vi "update_framescan.vi"(8 "error in (no error)":errorcluster, 9 "config cluster":T1={"DDS board initialization parameters"={"Bypass PLL"=FALSE, "PLL Range"=TRUE, "Update Clock"=FALSE, "Triangle "=FALSE, "SDO Active"=FALSE, "LSB First"=FALSE, "OSK Int"=FALSE, "Output Shaped Keying Enable"=TRUE, "Bypass Sinc"=FALSE, "Digital Part"=TRUE, "OutPut DAC"=TRUE, "Control DAC"=TRUE, "Comparator"=FALSE, "Modus"=0, "Multiplier Value"=15}, "OSK select"=TRUE, "inverse?"="normal", "AOD equilibration time"=0.0, "AOD amplitude"=0, "AOD center frequency"=0.0, "AOD Bandwidth"=0.0} {"DDS board initialization parameters"."Modus" scale=0.0..4.0}, 10 "settings cluster":T4={"number of pixels"=0, "maximum bit-depth"=0, "AOD center freq. (Hz)"=0.0, "AOD bandwidth freq. (Hz)"=0.0, "AOD amplitude"=0.0, "pixel dwell time"=0.0, "AOD equilibration time"=0.0, "x resolution"=0, "y resolution"=0, "z angle (rotation angle, phi)"=0.0, "x angle (tilting angle, phi)"=-1.0, "zoom"=-1.0, "channel offsets"={"channel 0"=0, "channel 1"=0, "channel 2"=0, "channel 3"=0}, "offset (Hz)"=[], "gates"=[], "enable clocks?"=FALSE}, 11 "FPGA VI Reference In":T3) -> (0 "error out":errorcluster)   [LabVIEW 2010]
doc: "This one is doing an update"
uses:
  FPGAWrapperMH120124FrameScan_PXI7813R/settings_cluster_framescan.ctl
  common_typedefs/channels_cluster.ctl
  fpgaVIsAndControls/gate_cluster.ctl
  common_typedefs/gate_parameters_cluster.ctl
  FPGAWrapperMH120124FrameScan_PXI7813R/FPGA_framescan_reference.ctl
  FPGAWrapperMH120124FrameScan_PXI7813R/configuration_cluster_framescan.ctl
  fpgaVIsAndControls/DDS_board_init_cluster.ctl
  <vilib>/rvi/interface/nirviReadWriteControl/nirviReadWriteControl.xnode
  <vilib>/rvi/interface/common/niFpgaNodeNameForErrorReporting.ctl
  <vilib>/rvi/errors/niLvFpgaWhatHappensToTopLevelVI.ctl
  <vilib>/Utility/error.llb/Error Cluster From Error Code.vi
  <vilib>/rvi/errors/niLvFpgaAdjustHostInterfaceError.vi
  NiFpgaLv.dll
panel:
  # "FSK"
  # "Ramped"
  # "FSK"
  # "Chirp Modus"
  # "Unramped"
  # "BPSK"
  # "Single Tone"
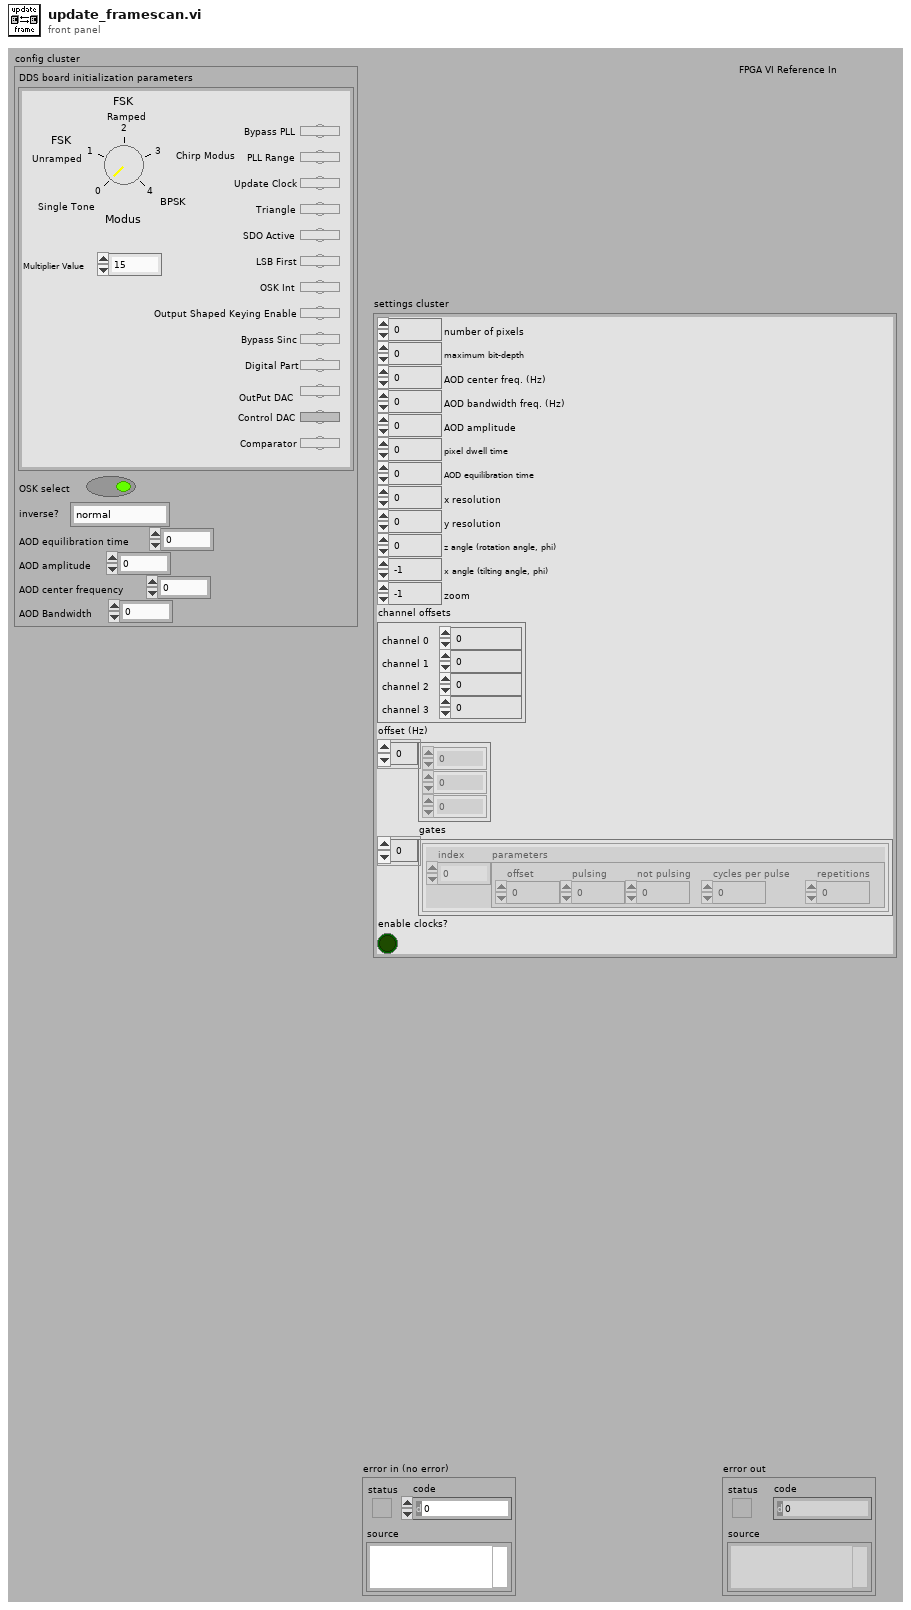
[diagram p1: front panel]
types:
  T1 = typedef "configuration_cluster_framescan.ctl" = cluster{"DDS board initialization parameters":T2, "OSK select":bool, "inverse?":string, "AOD equilibration time":dbl, "AOD amplitude":u16, "AOD center frequency":dbl, "AOD Bandwidth":dbl}
  T2 = typedef "DDS_board_init_cluster.ctl" = cluster{"Bypass PLL":bool, "PLL Range":bool, "Update Clock":bool, "Triangle ":bool, "SDO Active":bool, "LSB First":bool, "OSK Int":bool, "Output Shaped Keying Enable":bool, "Bypass Sinc":bool, "Digital Part":bool, "OutPut DAC":bool, "Control DAC":bool, "Comparator":bool, "Modus":u8, "Multiplier Value":u8}
  T3 = typedef "FPGA_framescan_reference.ctl" = refnum<k20>
  T4 = typedef "settings_cluster_framescan.ctl" = cluster{"number of pixels":i32, "maximum bit-depth":i8, "AOD center freq. (Hz)":dbl, "AOD bandwidth freq. (Hz)":dbl, "AOD amplitude":dbl, "pixel dwell time":dbl, "AOD equilibration time":dbl, "x resolution":i32, "y resolution":i32, "z angle (rotation angle, phi)":dbl, "x angle (tilting angle, phi)":dbl, "zoom":dbl, "channel offsets":T5, "offset (Hz)":dbl[], "gates":T6[], "enable clocks?":bool}
  T5 = typedef "channels_cluster.ctl" = cluster{"channel 0":u32, "channel 1":u32, "channel 2":u32, "channel 3":u32}
  T6 = typedef "gate_cluster.ctl" = cluster{"index":i32, "parameters":T7}
  T7 = typedef "gate_parameters_cluster.ctl" = cluster{"offset":i64, "pulsing":i64, "not pulsing":i64, "cycles per pulse":i64, "repetitions":i64}
  T8 = typedef "niFpgaNodeNameForErrorReporting.ctl" = enum16{"Open FPGA VI Reference", "Read/Write Control", "Invoke Method: Abort", "Invoke Method: Acknowledge IRQ", "Invoke Method: Download", "Invoke Method: FIFO.Configure", "Invoke Method: FIFO.Read", "Invoke Method: FIFO.Start", "Invoke Method: FIFO.Stop", "Invoke Method: FIFO.Write", "Invoke Method: Reset", "Invoke Method: Run", "Invoke Method: Wait on IRQ", "Close FPGA VI Reference"}
  T9 = typedef "niLvFpgaWhatHappensToTopLevelVI.ctl" = enum16{"top level VI scripted behind XNode", "top level VI inlined behind XNode"}
  T10 = cluster{"AOD Bandwidth_x (Hz)":fxp<+/-,36,32>, "AOD Bandwidth_y (Hz)":fxp<+/-,36,32>, "sin Phi":fxp<+/-,36,2>, "cos Phi":fxp<+/-,36,2>, "Bandwidth for LUTs (256pts)":fxp<+,36,0>, "AOD_Amplitude in":u16, "AOD center frequ. (Hz)_x":fxp<+/-,36,32>, "AOD center frequ. (Hz)_y":fxp<+/-,36,32>, "x offset (Hz)":fxp<+/-,36,32>, "y offset (Hz)":fxp<+/-,36,32>}
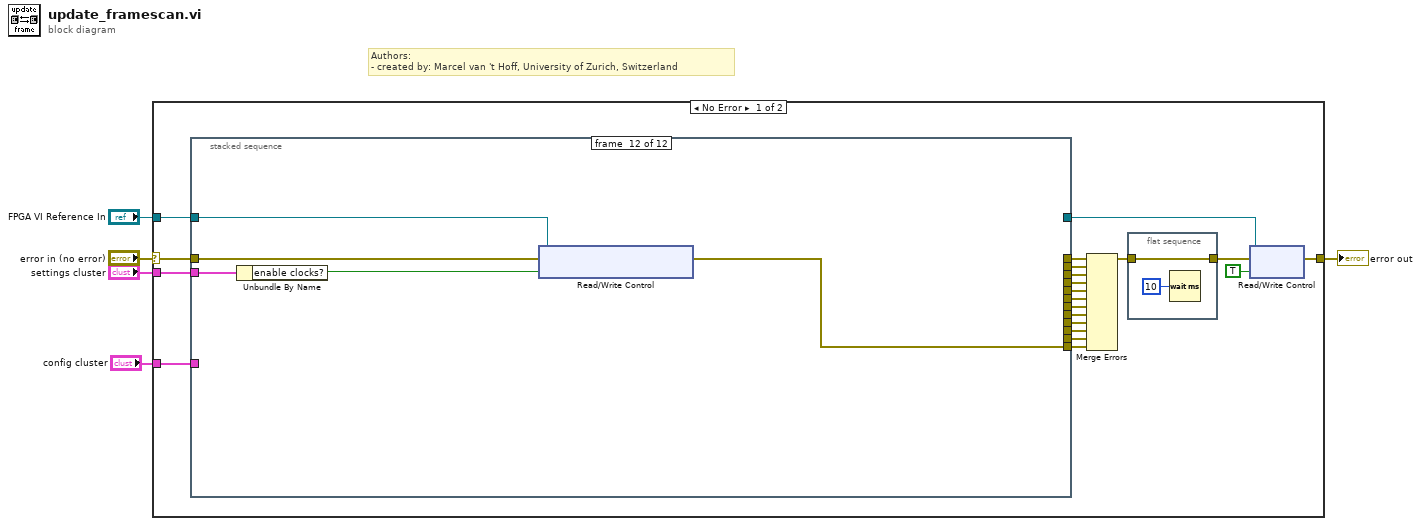
[diagram p0: block diagram]
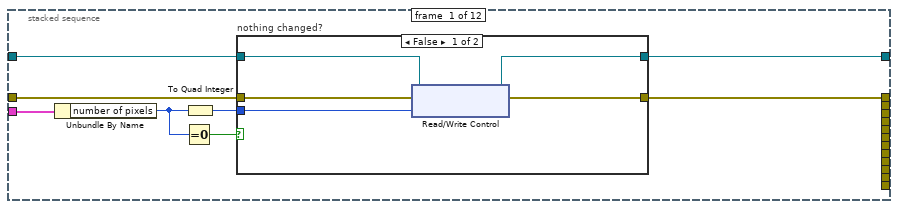
[diagram p2: hidden frame]
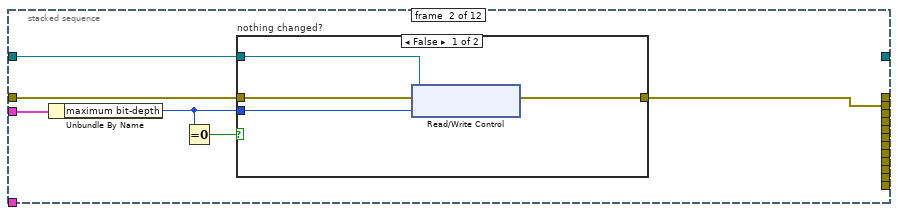
[diagram p4: hidden frame]
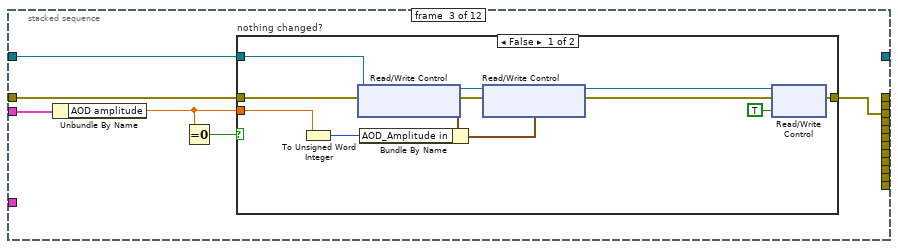
[diagram p6: hidden frame]
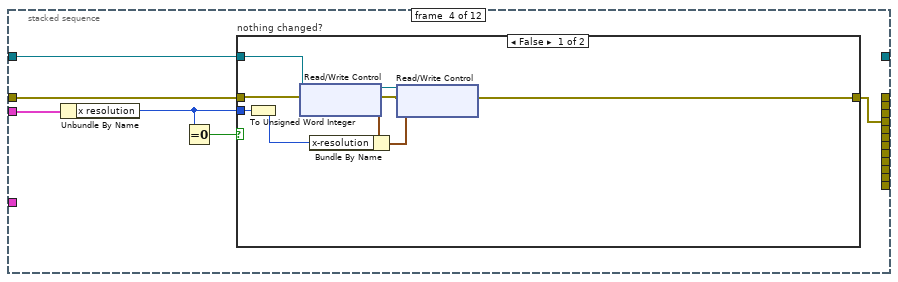
[diagram p8: hidden frame]
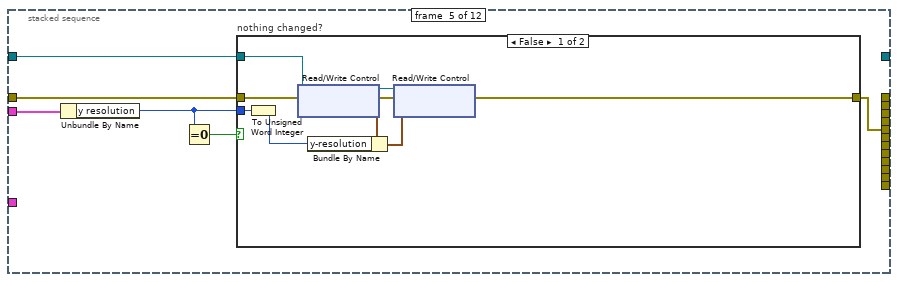
[diagram p10: hidden frame]
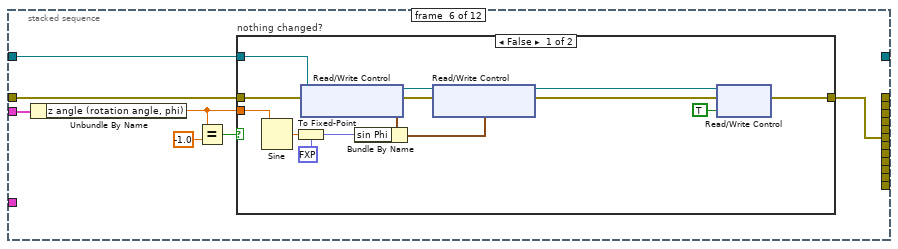
[diagram p12: hidden frame]
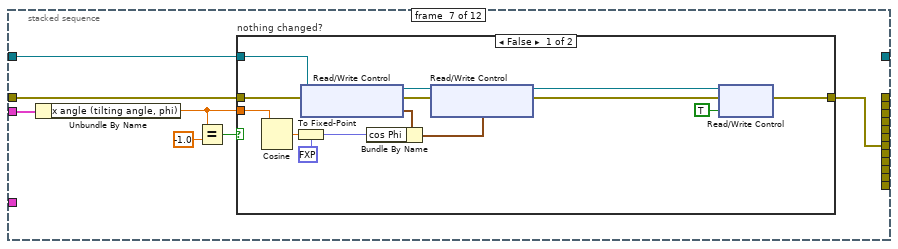
[diagram p14: hidden frame]
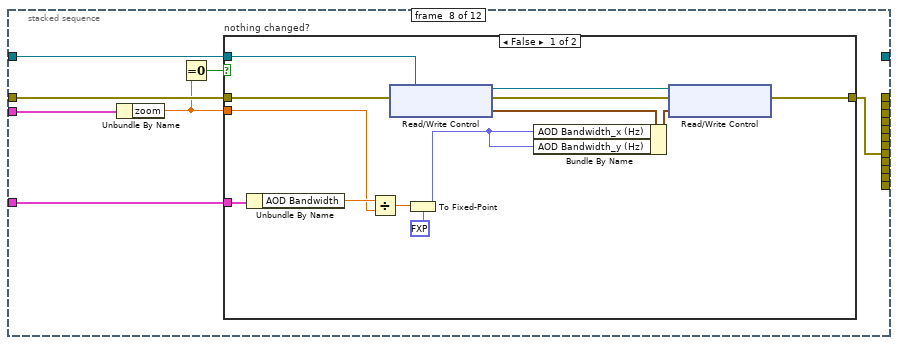
[diagram p16: hidden frame]
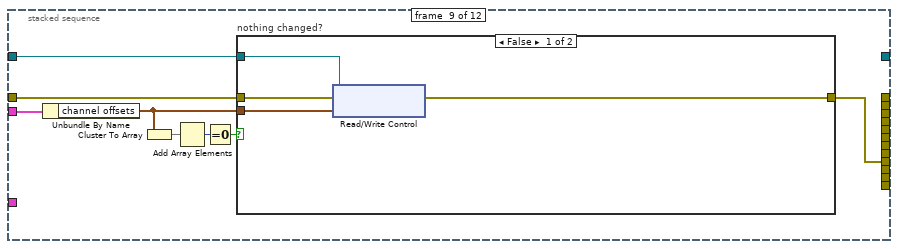
[diagram p18: hidden frame]
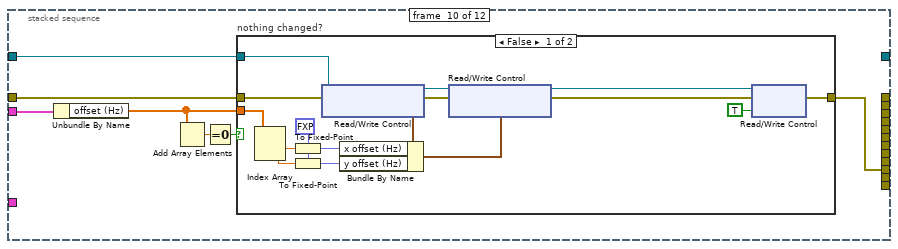
[diagram p20: hidden frame]
diagram:
  # "Authors: \n- created by: Marcel van 't Hoff, University of Zurich, Switzerland"
  n1 = case shown="No Error" "error in (no error)" {
    selector: "error in (no error)" -> [w13 w1389]
    tunnel: "settings cluster" -> [w12 _]
    tunnel: "FPGA VI Reference In" -> [w14 _]
    tunnel: [w25 w1389] -> w3
    tunnel: "config cluster" -> [w7 _]
    frame No Error {
      n2 = stacked-sequence {
        tunnel: w12 -> [w34 w91 w140 w292 w403 w515 w670 w825 w941 w997 w1152 w1308]
        tunnel: [w28 _ _ _ _ _ _ _ _ _ _ _] -> w15
        tunnel: w13 -> [w30 w89 w138 w290 w401 w514 w669 w824 w940 w996 w1149 w1307]
        tunnel: w14 -> [w29 w88 w137 w289 w400 w513 w668 w823 w939 w995 w1150 w1306]
        tunnel: [_ w86 _ _ _ _ _ _ _ _ _ _] -> w16
        tunnel: [_ _ w135 _ _ _ _ _ _ _ _ _] -> w17
        tunnel: [_ _ _ w287 _ _ _ _ _ _ _ _] -> w18
        tunnel: [_ _ _ _ w398 _ _ _ _ _ _ _] -> w19
        tunnel: [_ _ _ _ _ w509 _ _ _ _ _ _] -> w20
        tunnel: [_ _ _ _ _ _ w664 _ _ _ _ _] -> w21
        tunnel: [_ _ _ _ _ _ _ w820 _ _ _ _] -> w22
        tunnel: [_ _ _ _ _ _ _ _ w934 _ _ _] -> w23
        tunnel: [_ _ _ _ _ _ _ _ _ w991 _ _] -> w24
        tunnel: [w27 _ _ _ _ _ _ _ _ _ _ _] -> w10
        tunnel: [_ _ _ _ _ _ _ _ _ _ w1148 _] -> w9
        tunnel: w7 -> [_ _ _ _ _ _ _ w819 _ _ _ _]
        tunnel: [_ _ _ _ _ _ _ _ _ _ _ w1305] -> w6
        frame #0 {
          n3 = Unbundle By Name(w34) -> ("number of pixels"=w33:i32)
          n4 = Equal To 0?(x=w33) -> (x = 0?=w32:bool)
          n5 = To Quad Integer(1:w33) -> (0:w31:i64)
          n6 = case "nothing changed?" shown="False" w32 {
            tunnel: w31 -> [w37 _]
            tunnel: [w39 w85] -> w28
            tunnel: w30 -> [w38 w85]
            tunnel: w29 -> [w36 w84]
            tunnel: [w35 w84] -> w27
            frame False {
              n7 = xnode "Read/Write Control"("FPGA VI Reference In"=w36, "error in"=w38, "number of pixels"=w37) -> ("FPGA VI Reference Out"=w35:T3, "error out"=w39:errorcluster)
            }
            frame True {
              # "nothing changed"
            }
          }
        }
        frame #1 {
          n8 = Unbundle By Name(w91) -> ("maximum bit-depth"=w87:i8)
          n9 = Equal To 0?(x=w87) -> (x = 0?=w90:bool)
          n10 = case "nothing changed?" shown="False" w90 {
            tunnel: w87 -> [w93 _]
            tunnel: [w95 w134] -> w86
            tunnel: w89 -> [w94 w134]
            tunnel: w88 -> [w92 _]
            frame False {
              n11 = xnode "Read/Write Control"("FPGA VI Reference In"=w92, "error in"=w94, "maximum bit depth"=w93) -> ("error out"=w95:errorcluster)  [unwired: 1 out]
            }
            frame True {
              # "nothing changed"
            }
          }
        }
        frame #2 {
          n12 = Unbundle By Name(w140) -> ("AOD amplitude"=w136:dbl)
          n13 = Equal To 0?(x=w136) -> (x = 0?=w139:bool)
          n14 = case "nothing changed?" shown="False" w139 {
            tunnel: [w145 w286] -> w135
            tunnel: w138 -> [w150 w286]
            tunnel: w137 -> [w152 _]
            tunnel: w136 -> [w148 _]
            frame False {
              n15 = To Unsigned Word Integer(number=w148) -> (unsigned 16bit integer=w147:u16)
              n16 = xnode "Read/Write Control"("FPGA VI Reference In"=w152, "error in"=w150) -> ("FPGA VI Reference Out"=w151:T3, "error out"=w149:errorcluster, "FPGA parameters"=w142:T10)
              n17 = Bundle By Name(cluster=w142, "AOD_Amplitude in"=w147) -> (w141:T10)
              n18 = xnode "Read/Write Control"("FPGA VI Reference In"=w151, "error in"=w149, "FPGA parameters"=w141) -> ("FPGA VI Reference Out"=w144:T3, "error out"=w146:errorcluster)
              n19 = xnode "Read/Write Control"("FPGA VI Reference In"=w144, "error in"=w146, "reset in"=TRUE) -> ("error out"=w145:errorcluster)  [unwired: 1 out]
            }
            frame True {
              # "nothing changed"
            }
          }
        }
        frame #3 {
          n20 = Unbundle By Name(w292) -> ("x resolution"=w288:i32)
          n21 = Equal To 0?(x=w288) -> (x = 0?=w291:bool)
          n22 = case "nothing changed?" shown="False" w291 {
            tunnel: [w295 w397] -> w287
            tunnel: w290 -> [w298 w397]
            tunnel: w289 -> [w297 _]
            tunnel: w288 -> [w301 _]
            frame False {
              n23 = To Unsigned Word Integer(number=w301) -> (unsigned 16bit integer=w296:u16)
              n24 = xnode "Read/Write Control"("FPGA VI Reference In"=w297, "error in"=w298) -> ("FPGA VI Reference Out"=w293:T3, "error out"=w294:errorcluster, "scan settings"=w300:cluster{"x-resolution":u16, "y-resolution":u16})
              n25 = Bundle By Name(cluster=w300, "x-resolution"=w296) -> (w299:cluster{"x-resolution":u16, "y-resolution":u16})
              n26 = xnode "Read/Write Control"("FPGA VI Reference In"=w293, "error in"=w294, "scan settings"=w299) -> ("error out"=w295:errorcluster)  [unwired: 1 out]
            }
            frame True {
              # "nothing changed"
            }
          }
        }
        frame #4 {
          n27 = Unbundle By Name(w403) -> ("y resolution"=w399:i32)
          n28 = Equal To 0?(x=w399) -> (x = 0?=w402:bool)
          n29 = case "nothing changed?" shown="False" w402 {
            tunnel: [w408 w508] -> w398
            tunnel: w401 -> [w410 w508]
            tunnel: w400 -> [w411 _]
            tunnel: w399 -> [w412 _]
            frame False {
              n30 = To Unsigned Word Integer(number=w412) -> (unsigned 16bit integer=w405:u16)
              n31 = xnode "Read/Write Control"("FPGA VI Reference In"=w411, "error in"=w410) -> ("FPGA VI Reference Out"=w407:T3, "error out"=w409:errorcluster, "scan settings"=w406:cluster{"x-resolution":u16, "y-resolution":u16})
              n32 = Bundle By Name(cluster=w406, "y-resolution"=w405) -> (w404:cluster{"x-resolution":u16, "y-resolution":u16})
              n33 = xnode "Read/Write Control"("FPGA VI Reference In"=w407, "error in"=w409, "scan settings"=w404) -> ("error out"=w408:errorcluster)  [unwired: 1 out]
            }
            frame True {
              # "nothing changed"
            }
          }
        }
        frame #5 {
          n34 = Unbundle By Name(w515) -> ("z angle (rotation angle, phi)"=w512:dbl)
          n35 = Equal?(x=w512, y=-1.0) -> (x = y?=w511:bool)
          n36 = case "nothing changed?" shown="False" w511 {
            tunnel: [w519 w663] -> w509
            tunnel: w514 -> [w524 w663]
            tunnel: w513 -> [w526 _]
            tunnel: w512 -> [w529 _]
            frame False {
              n37 = Sine(x=w529) -> (sin(x)=w527:dbl)
              n38 = To Fixed-Point(fixed-point type=fxp<+/-,36,2> 0.0 ("sin Phi"), number=w527) -> (fixed-point=w522:fxp<+/-,36,2>)
              n39 = xnode "Read/Write Control"("FPGA VI Reference In"=w526, "error in"=w524) -> ("FPGA VI Reference Out"=w525:T3, "error out"=w523:errorcluster, "FPGA parameters"=w517:T10)
              n40 = Bundle By Name(cluster=w517, "sin Phi"=w522) -> (w516:T10)
              n41 = xnode "Read/Write Control"("FPGA VI Reference In"=w525, "error in"=w523, "FPGA parameters"=w516) -> ("FPGA VI Reference Out"=w520:T3, "error out"=w521:errorcluster)
              n42 = xnode "Read/Write Control"("FPGA VI Reference In"=w520, "error in"=w521, "reset in"=TRUE) -> ("error out"=w519:errorcluster)  [unwired: 1 out]
            }
            frame True {
              # "nothing changed"
            }
          }
        }
        frame #6 {
          n43 = Unbundle By Name(w670) -> ("x angle (tilting angle, phi)"=w667:dbl)
          n44 = Equal?(x=w667, y=-1.0) -> (x = y?=w666:bool)
          n45 = case "nothing changed?" shown="False" w666 {
            tunnel: [w674 w818] -> w664
            tunnel: w669 -> [w679 w818]
            tunnel: w668 -> [w681 _]
            tunnel: w667 -> [w684 _]
            frame False {
              n46 = Cosine(x=w684) -> (cos(x)=w682:dbl)
              n47 = To Fixed-Point(fixed-point type=fxp<+/-,36,2> 0.0 ("sin Phi"), number=w682) -> (fixed-point=w677:fxp<+/-,36,2>)
              n48 = xnode "Read/Write Control"("FPGA VI Reference In"=w681, "error in"=w679) -> ("FPGA VI Reference Out"=w680:T3, "error out"=w678:errorcluster, "FPGA parameters"=w673:T10)
              n49 = Bundle By Name(cluster=w673, "cos Phi"=w677) -> (w672:T10)
              n50 = xnode "Read/Write Control"("FPGA VI Reference In"=w680, "error in"=w678, "FPGA parameters"=w672) -> ("FPGA VI Reference Out"=w675:T3, "error out"=w676:errorcluster)
              n51 = xnode "Read/Write Control"("FPGA VI Reference In"=w675, "error in"=w676, "reset in"=TRUE) -> ("error out"=w674:errorcluster)  [unwired: 1 out]
            }
            frame True {
              # "nothing changed"
            }
          }
        }
        frame #7 {
          n52 = Unbundle By Name(w825) -> ("zoom"=w822:dbl)
          n53 = Equal To 0?(x=w822) -> (x = 0?=w821:bool)
          n54 = case "nothing changed?" shown="False" w821 {
            tunnel: [w832 w933] -> w820
            tunnel: w824 -> [w836 w933]
            tunnel: w823 -> [w838 _]
            tunnel: w822 -> [w828 _]
            tunnel: w819 -> [w830 _]
            frame False {
              n55 = Unbundle By Name(w830) -> ("AOD Bandwidth"=w829:dbl)
              n56 = Divide(x=w829, y=w828) -> (x/y=w827:dbl)
              n57 = xnode "Read/Write Control"("FPGA VI Reference In"=w838, "error in"=w836) -> ("FPGA VI Reference Out"=w837:T3, "error out"=w835:errorcluster, "FPGA parameters"=w831:T10)
              n58 = To Fixed-Point(fixed-point type=fxp<+/-,36,32> 1.0 ("AOD_Scale_Factor (1/Zoom)"), number=w827) -> (fixed-point=w826:fxp<+/-,36,32>)
              n59 = Bundle By Name(cluster=w831, "AOD Bandwidth_x (Hz)"=w826, "AOD Bandwidth_y (Hz)"=w826) -> (w833:T10)
              n60 = xnode "Read/Write Control"("FPGA VI Reference In"=w837, "error in"=w835, "FPGA parameters"=w833) -> ("error out"=w832:errorcluster)  [unwired: 1 out]
            }
            frame True {
              # "nothing changed"
            }
          }
        }
        frame #8 {
          n61 = Unbundle By Name(w941) -> ("channel offsets"=w938:T5)
          n62 = Cluster To Array(cluster=w938) -> (array=w936:u32[])
          n63 = Add Array Elements(numeric array=w936) -> (sum=w935:u32)
          n64 = Equal To 0?(x=w935) -> (x = 0?=w937:bool)
          n65 = case "nothing changed?" shown="False" w937 {
            tunnel: [w943 w990] -> w934
            tunnel: w940 -> [w944 w990]
            tunnel: w939 -> [w945 _]
            tunnel: w938 -> [w942 _]
            frame False {
              n66 = xnode "Read/Write Control"("FPGA VI Reference In"=w945, "error in"=w944, "channel offsets"=w942) -> ("error out"=w943:errorcluster)  [unwired: 1 out]
            }
            frame True {
              # "nothing changed"
            }
          }
        }
        frame #9 {
          n67 = Unbundle By Name(w997) -> ("offset (Hz)"=w992:dbl[])
          n68 = Add Array Elements(numeric array=w992) -> (sum=w993:dbl)
          n69 = Equal To 0?(x=w993) -> (x = 0?=w994:bool)
          n70 = case "nothing changed?" shown="False" w994 {
            tunnel: [w1001 w1147] -> w991
            tunnel: w996 -> [w1012 w1147]
            tunnel: w995 -> [w1013 _]
            tunnel: w992 -> [w1010 _]
            frame False {
              w1011 = fxp<+/-,36,32> 0.0 ("x offset (Hz)")
              n71 = Index Array(array=w1010) -> (element #1=w1009:dbl, element #2=w1008:dbl)  [unwired: 2 in]
              n72 = To Fixed-Point(fixed-point type=w1011, number=w1009) -> (fixed-point=w1005:fxp<+/-,36,32>)
              n73 = To Fixed-Point(fixed-point type=w1011, number=w1008) -> (fixed-point=w1004:fxp<+/-,36,32>)
              n74 = xnode "Read/Write Control"("FPGA VI Reference In"=w1013, "error in"=w1012) -> ("FPGA VI Reference Out"=w1007:T3, "error out"=w1006:errorcluster, "FPGA parameters"=w1000:T10)
              n75 = Bundle By Name(cluster=w1000, "x offset (Hz)"=w1005, "y offset (Hz)"=w1004) -> (w999:T10)
              n76 = xnode "Read/Write Control"("FPGA VI Reference In"=w1007, "error in"=w1006, "FPGA parameters"=w999) -> ("FPGA VI Reference Out"=w1002:T3, "error out"=w1003:errorcluster)
              n77 = xnode "Read/Write Control"("FPGA VI Reference In"=w1002, "error in"=w1003, "reset in"=TRUE) -> ("error out"=w1001:errorcluster)  [unwired: 1 out]
            }
            frame True {
              # "nothing changed"
            }
          }
        }
        frame #10 {
          n78 = Unbundle By Name(w1152) -> ("gates"=w1151:T6[])
          n79 = for "Loop over specified gates..." {
            tunnel: w1151 -> [w1158] mode=indexing
            tunnel: w1150 -> [w1157]
            shift-right: [w1155] -> w1148
            shift-left: w1149 -> [w1156]
            stop <- w1155 stop-if-true
            n80 = Unbundle By Name(w1158) -> ("index"=w1153:i32, "parameters"=w1154:T7)
            n81 = case "Which gate?" shown="1" w1153 {
              tunnel: w1157 -> [_ w1163 w1209 w1259]
              tunnel: w1156 -> [w1159 w1162 w1211 w1258]
              tunnel: [w1159 w1161 w1210 w1257] -> w1155
              tunnel: w1154 -> [_ w1160 w1208 w1256]
              frame Default {
              }
              frame 1 {
                n82 = xnode "Read/Write Control"("FPGA VI Reference In"=w1163, "error in"=w1162, "gate 1"=w1160) -> ("error out"=w1161:errorcluster)  [unwired: 1 out]
              }
              frame 2 {
                n83 = xnode "Read/Write Control"("FPGA VI Reference In"=w1209, "error in"=w1211, "gate 2"=w1208) -> ("error out"=w1210:errorcluster)  [unwired: 1 out]
              }
              frame 3 {
                n84 = xnode "Read/Write Control"("FPGA VI Reference In"=w1259, "error in"=w1258, "gate 3"=w1256) -> ("error out"=w1257:errorcluster)  [unwired: 1 out]
              }
            }
          }
        }
        frame #11 {
          n85 = Unbundle By Name(w1308) -> ("enable clocks?"=w1304:bool)
          n86 = xnode "Read/Write Control"("FPGA VI Reference In"=w1306, "error in"=w1307, "shall acquisition start clocks?"=w1304) -> ("error out"=w1305:errorcluster)  [unwired: 1 out]
        }
      }
      n87 = Merge Errors(w15, w16, w17, w18, w19, w20, w21, w22, w23, w24, w9, w6) -> (w11:errorcluster)
      n88 = flat-sequence {
        tunnel: [w1348] -> w26
        tunnel: w11 -> [w1348]
        frame #0 {
          n89 = Wait (ms)(milliseconds to wait=u32 10) -> ()  [unwired: 1 out]
        }
      }
      n90 = xnode "Read/Write Control"("FPGA VI Reference In"=w10, "error in"=w26, "reset in"=TRUE) -> ("error out"=w25:errorcluster)  [unwired: 1 out]
    }
    frame Error {
    }
  }
  "error out" <- w3
